vi "송신수신02.vi"() -> ()   [LabVIEW 2014]
panel:
  in  "정지":bool
  out "데이터 출력":string
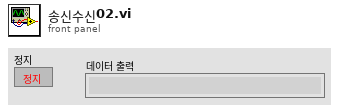
[diagram p1: front panel]
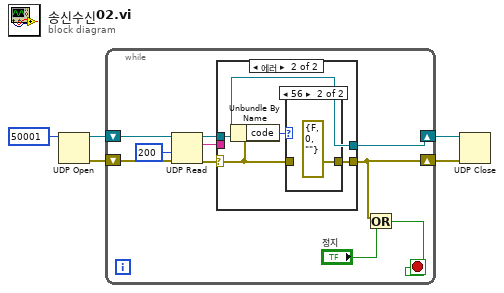
[diagram p0: block diagram]
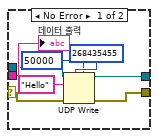
[diagram p2: hidden frame]
diagram:
  n1 = UDP Open(11:u16 50001 ("포트")) -> (port=w5:refnum<k16>, 0:w3:errorcluster)  [unwired: 4 in, 1 out]
  n2 = while {
    shift-right: [w6] -> w4
    shift-left: w5 -> [w15]
    shift-right: [w8] -> w2
    shift-left: w3 -> [w14]
    stop <- w12 stop-if-true
    n3 = UDP Read(connection ID=w15, timeout ms (25000)=200 ("타임아웃 ms (25000)"), 8:w14) -> (data out=w13:string, error out=w9:errorcluster, 3:w7:refnum<k16>)  [unwired: 1 in, 2 out]
    n4 = case shown="에러" w9 {
      selector: w9 -> [w20 w25]
      tunnel: w13 -> [w23 _]
      tunnel: [w19 w26] -> w8
      tunnel: w7 -> [w18 w24]
      tunnel: [w17 w24] -> w6
      frame No Error {
        n5 = UDP Write(address=u32 268435455 ("주소"), port or service name=u16 50000 ("포트 또는 서비스 이름"), connection ID=w18, data in="Hello" ("데이터 입력"), 8:w20) -> (error out=w19:errorcluster, 3:w17:refnum<k16>)  [unwired: 1 in]
        "데이터 출력" <- w23
      }
      frame Error {
        n6 = Unbundle By Name(w25) -> ("code"=w27:i32)
        n7 = case shown="56" w27 {
          tunnel: [w28 errorcluster {"status"=FALSE, "code"=0, "source"=""} ("에러 상수")] -> w26
          tunnel: w25 -> [w28 _]
          frame Default {
          }
          frame 56 {
          }
        }
      }
    }
    n8 = Or(x=w8, y="정지") -> (x .or. y?=w12:bool)
  }
  n9 = UDP Close(connection ID=w4, 8:w2) -> ()  [unwired: 2 out]
